vi "Read Arr of Channel Ref.vi"(8 "error in (no error)":errorcluster, 11 "Generic Data Logger Card in":refnum<class "Generic Data Logger Card.lvclass">) -> (0 "error out":errorcluster, 2 "Arr of Channel Ref":refnum<vi>, 3 "Generic Data Logger Card out":refnum<class "Generic Data Logger Card.lvclass">)   [LabVIEW 2013, in "Generic Data Logger.lvlib" / "Generic Data Logger Card.lvclass"]
uses:
  Generic Data Logger Card.lvclass
  Generic Data Logger Card.lvclass/Generic Data Logger Card.ctl
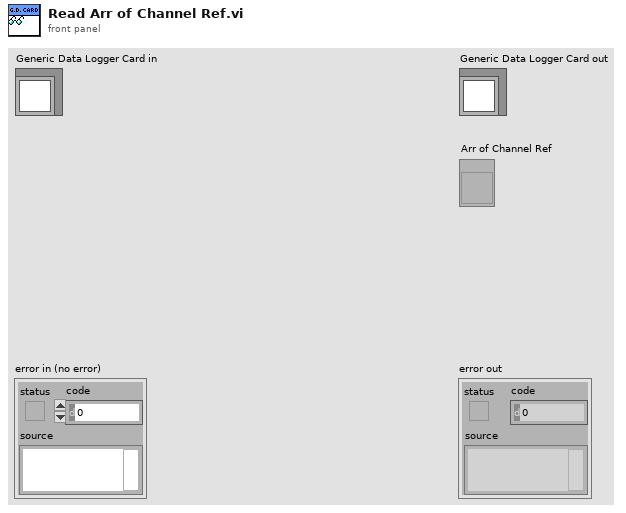
[diagram p1: front panel]
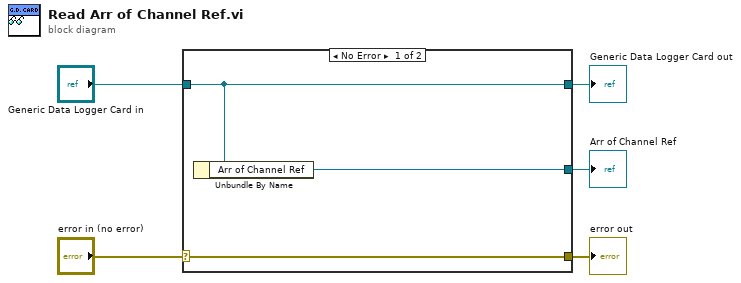
[diagram p0: block diagram]
diagram:
  n1 = case shown="No Error" "error in (no error)" {
    selector: "error in (no error)" -> [w8 w9]
    tunnel: [w8 w9] -> w4
    tunnel: [w7 w10] -> w2
    tunnel: "Generic Data Logger Card in" -> [w7 w10]
    tunnel: [w6 _] -> w1
    frame No Error {
      n2 = Unbundle By Name(w7) -> ("Arr of Channel Ref"=w6:refnum<vi>)
    }
    frame Error {
    }
  }
  "error out" <- w4
  "Generic Data Logger Card out" <- w2
  "Arr of Channel Ref" <- w1
